vi "Autonomous.vi"   [LabVIEW 2020]
doc: "This VI starts when autonomous period begins, and will automatically be terminated when it ends. You can carry out timed or sensor driven operations directly to I/O or to subsystems without needing to return to the caller."
uses:
  <vilib>/Rock Robotics/WPI/Utilities/WPI_GetSetVariantRefNum.vi
  <vilib>/Rock Robotics/Network Tables/NT Read String.vi
types:
  T1 = typedef "WPI_JoystickDevRef.ctl" = cluster{"Device":T2}
  T2 = typedef "WPI_JoystickDeviceEnum.ctl" = enum16{"USB 0", "USB 1", "USB 2", "USB 3", "USB 4", "USB 5"}
  T3 = typedef "Command Status Info.ctl" = cluster{"Name":string, "Status":T4, "notifier out":T5}
  T4 = typedef "Completion Status.ctl" = enum16{"Successful", "Aborted", "Incomplete"}
  T5 = typedef "Completion Notifier.ctl" = refnum<notifier>
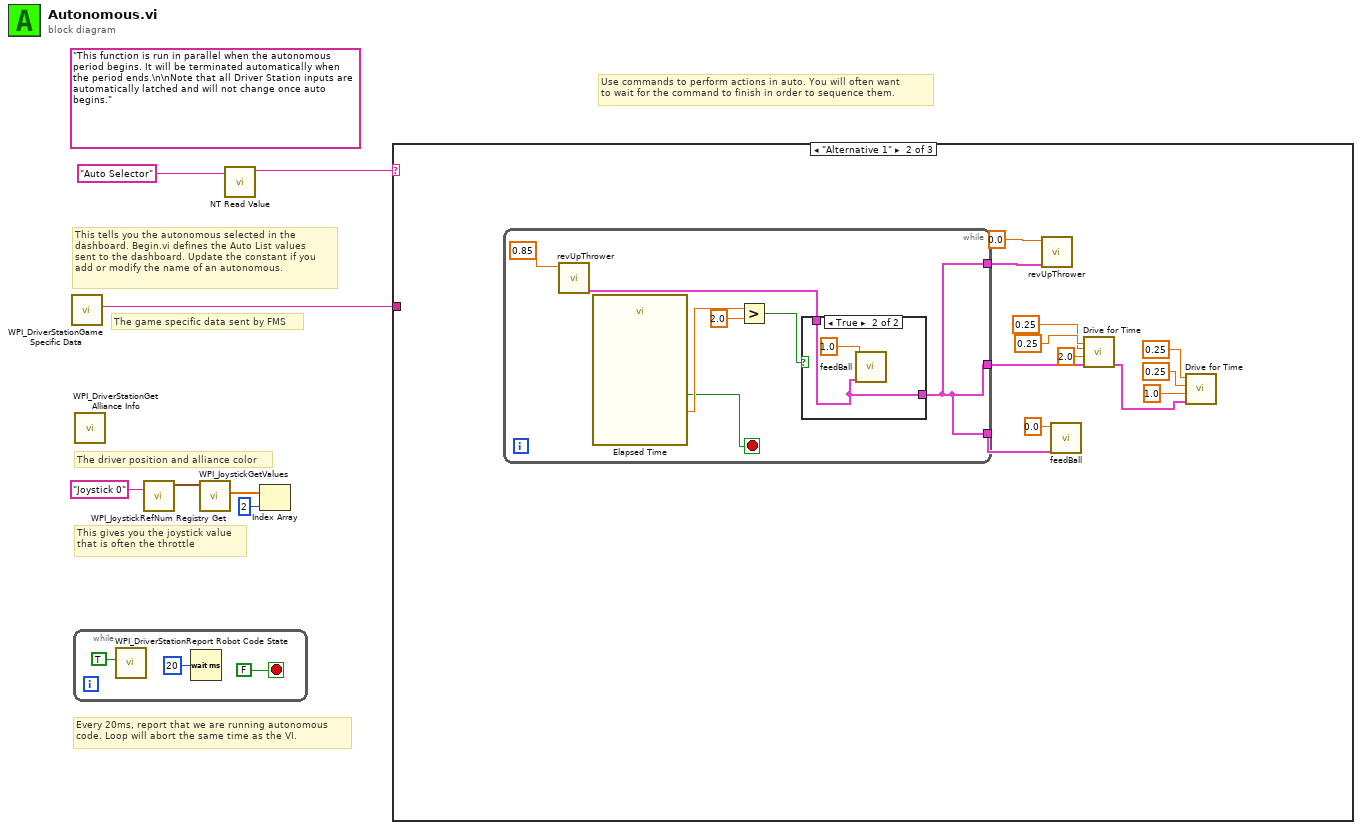
[diagram p0: block diagram]
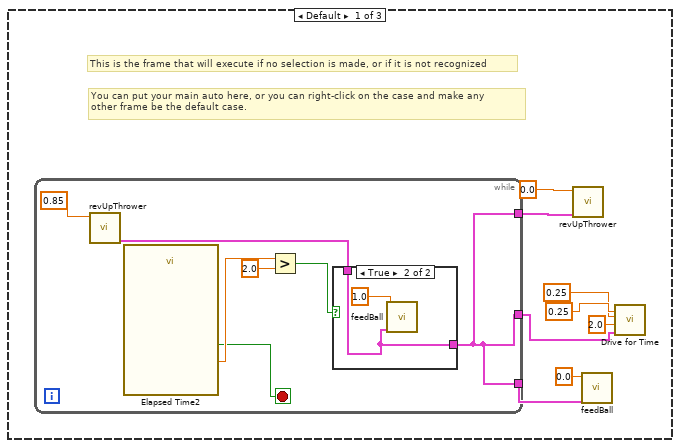
[diagram p2: hidden frame]
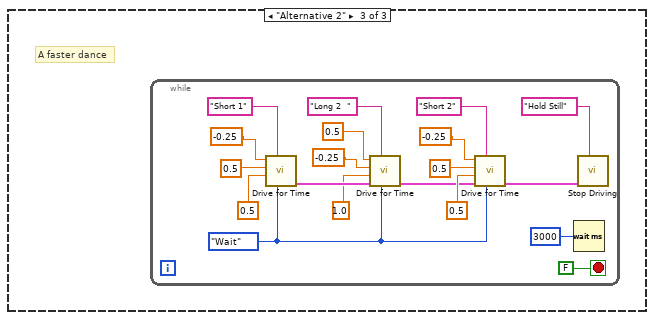
[diagram p5: hidden frame]
diagram:
  (unwired) "This function is run in parallel when the autonomous period begins. It will be terminated automatically when the period ends.\n\nNote that all Driver Station inputs are automatically latched and will not change once auto begins."
  # "The game specific data sent by FMS"
  # "This tells you the autonomous selected in the \ndashboard. Begin.vi defines the Auto List values\nsent to the dashboard. Update the constant if you\nadd or modify the name of an autonomous."
  # "Every 20ms, report that we are running autonomous\ncode. Loop will abort the same time as the VI."
  # "This gives you the joystick value\nthat is often the throttle"
  # "Use commands to perform actions in auto. You will often want\nto wait for the command to finish in order to sequence them."
  # "The driver position and alliance color"
  n1 = call <vilib>:"WPI_DriverStationGame Specific Data.vi"() -> ("Game Specific Data"=w1:string)  [unwired: 11 in]
  n2 = while {
    stop <- FALSE stop-if-true
    n3 = call <vilib>:"WPI_DriverStationReport Robot Code State.vi"("Autonomous"=TRUE) -> ()  [unwired: 10 in, 1 out]
    n4 = Wait (ms)(milliseconds to wait=u32 20) -> ()  [unwired: 1 out]
  }
  n5 = call <vilib>:"WPI_DriverStationGet Alliance Info.vi"() -> ()  [unwired: 12 out]
  n6 = call <vilib>:"WPI_JoystickRefNum Registry Get.vi"("refnum name"="Joystick 0") -> ("JoystickDevRef"=w6:T1)  [unwired: 1 in, 9 out]
  n7 = call <vilib>:"WPI_JoystickGetValues.vi"("JoystickDevRef"=w6) -> ("Axes"=w5:dbl[])  [unwired: 6 in, 4 out]
  n8 = call-poly <vilib>:"NT Read Value.vi"("Name"="Auto Selector") -> ("String"=w2:string)  [unwired: 9 in, 1 out]
  n9 = Index Array(array=w5, index=2) -> ()  [unwired: 1 out]
  n10 = case shown="\"Alternative 1\"" w2 {
    tunnel: w1 -> [_ _ _]
    frame Default {
      # "You can put your main auto here, or you can right-click on the case and make any\nother frame be the default case."
      # "This is the frame that will execute if no selection is made, or if it is not recognized"
      n11 = while {
        tunnel: [w19] -> w15
        tunnel: [w19] -> w14
        tunnel: [w19] -> w12
        stop <- w21 stop-if-true
        n12 = call "revUpThrower.vi"("Setpoint"=0.85) -> ("Command Info Out"=w20:T3)  [unwired: 10 in]
        n13 = call "Elapsed Time2"() -> ("Elapsed Time (s)"=w24:dbl, "Time has Elapsed"=w21:bool)  [unwired: 12 in, 6 out]
        n14 = Greater?(x=w24, y=2.0) -> (0:w22:bool)
        n15 = case shown="True" w22 {
          tunnel: w20 -> [_ w26]
          tunnel: [_ w26] -> w19
          frame False {
          }
          frame True {
            n16 = call "feedBall.vi"("Command Info In"=w26, "Setpoint"=1.0) -> ()  [unwired: 9 in, 1 out]
          }
        }
      }
      n17 = call "revUpThrower.vi"("Command Info In"=w14, "Setpoint"=0.0) -> ()  [unwired: 9 in, 1 out]
      n18 = call "feedBall.vi"("Command Info In"=w12, "Setpoint"=0.0) -> ()  [unwired: 9 in, 1 out]
      n19 = call "Drive for Time.vi"("Command Info In"=w15, "Seconds"=2.0, "Right Speed"=0.25, "Left Speed"=0.25) -> ()  [unwired: 7 in, 1 out]
    }
    frame "Alternative 1" {
      n20 = while {
        tunnel: [w40] -> w36
        tunnel: [w40] -> w35
        tunnel: [w40] -> w33
        stop <- w42 stop-if-true
        n21 = call "revUpThrower.vi"("Setpoint"=0.85) -> ("Command Info Out"=w41:T3)  [unwired: 10 in]
        n22 = call "Elapsed Time"() -> ("Elapsed Time (s)"=w45:dbl, "Time has Elapsed"=w42:bool)  [unwired: 12 in, 6 out]
        n23 = Greater?(x=w45, y=2.0) -> (0:w43:bool)
        n24 = case shown="True" w43 {
          tunnel: w41 -> [_ w47]
          tunnel: [_ w47] -> w40
          frame False {
          }
          frame True {
            n25 = call "feedBall.vi"("Command Info In"=w47, "Setpoint"=1.0) -> ()  [unwired: 9 in, 1 out]
          }
        }
      }
      n26 = call "revUpThrower.vi"("Command Info In"=w35, "Setpoint"=0.0) -> ()  [unwired: 9 in, 1 out]
      n27 = call "feedBall.vi"("Command Info In"=w33, "Setpoint"=0.0) -> ()  [unwired: 9 in, 1 out]
      n28 = call "Drive for Time.vi"("Command Info In"=w36, "Seconds"=2.0, "Right Speed"=0.25, "Left Speed"=0.25) -> ("Command Info Out"=w31:T3)  [unwired: 7 in]
      n29 = call "Drive for Time.vi"("Command Info In"=w31, "Seconds"=1.0, "Right Speed"=0.25, "Left Speed"=0.25) -> ()  [unwired: 7 in, 1 out]
    }
    frame "Alternative 2" {
      # "A faster dance"
      n30 = while {
        stop <- FALSE stop-if-true
        w49 = enum16{"Start", "Wait"}."Wait" ("Synchronication")
        n31 = call "Drive for Time.vi"("Synchronization"=w49, "Description"="Short 1", "Seconds"=0.5 ("Delay (s)"), "Right Speed"=0.5 ("X axis value"), "Left Speed"=-0.25 ("X axis value")) -> ("Command Info Out"=w67:T3)  [unwired: 6 in]
        n32 = call "Drive for Time.vi"("Synchronization"=w49, "Description"="Long 2  ", "Command Info In"=w67, "Seconds"=1.0 ("Delay (s)"), "Right Speed"=-0.25 ("X axis value"), "Left Speed"=0.5 ("X axis value")) -> ("Command Info Out"=w51:T3)  [unwired: 5 in]
        n33 = call "Drive for Time.vi"("Synchronization"=w49, "Description"="Short 2", "Command Info In"=w51, "Seconds"=0.5 ("Delay (s)"), "Right Speed"=0.5 ("X axis value"), "Left Speed"=-0.25 ("X axis value")) -> ("Command Info Out"=w50:T3)  [unwired: 5 in]
        n34 = Wait (ms)(milliseconds to wait=u32 3000 ("millisecond timer value")) -> ()  [unwired: 1 out]
        n35 = call "Stop Driving.vi"("Description"="Hold Still", "Command Info In"=w50) -> ()  [unwired: 9 in, 1 out]
      }
    }
  }
